vi "TH_LoggLine.vi"(6 "Händelse Logg In":string, 7 "Logg String In":string) -> (3 "Händelse Logg Out":string)   [LabVIEW 2014]
panel:
  out "Path":path
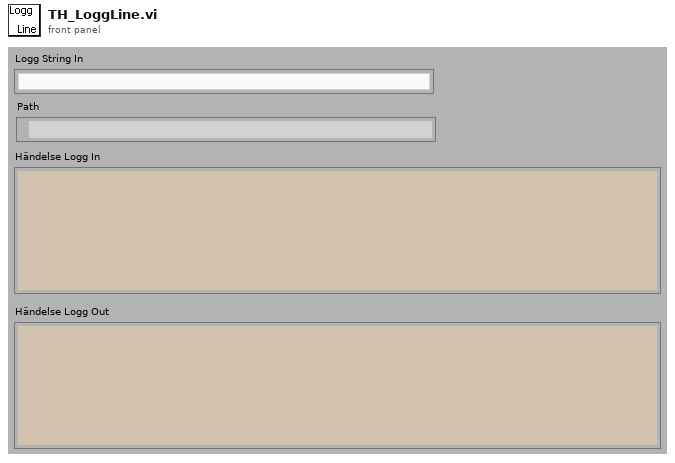
[diagram p1: front panel]
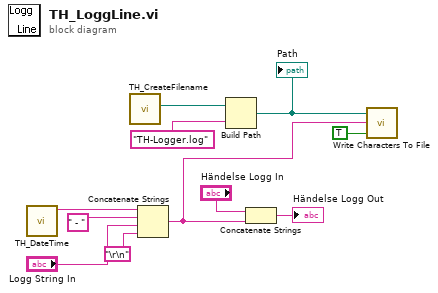
[diagram p0: block diagram]
diagram:
  n1 = call "TH_DateTime.vi"() -> ("Tid och Datum"=w11:string)  [unwired: 7 in]
  n2 = call "TH_CreateFilename.vi"() -> ("RootPath"=w1:path)  [unwired: 5 in, 2 out]
  n3 = Concatenate Strings(w11, " - " ("Substring"), "Logg String In", "\r\n") -> (w3:string)
  n4 = Build Path(base path=w1, name or relative path="TH-Logger.log") -> (appended path=w6:path)
  "Path" <- w6
  n5 = Concatenate Strings("Händelse Logg In", w3) -> (→"Händelse Logg Out":string)
  n6 = call <vilib>:"Write Characters To File.vi"("append to file? (new file:F)"=TRUE, "character string"=w3, "file path (dialog if empty)"=w6) -> ()  [unwired: 2 in, 1 out]
